vi "Configure Line Synchronization.vi"(6 "Enable Line Sync (F: Disable)":bool, 8 "error in (no error)":errorcluster, 9 "Channel List(\"\")":string, 10 "Function (0: Voltage DC)":i32(ring) items=[" Voltage DC"=0, "Current DC"=2, "Resistance"=4, "4-wire resistance"=5, "Temperature"=8, "Continuity"=9, "Voltage Ratio"=12], 11 "VISA resource name":refnum<visa-resource-name>) -> (0 "error out":errorcluster, 3 "VISA resource name out":refnum<visa-resource-name>)   [LabVIEW 2020, in "Keithley DMM6500 DAQ6500 Series.lvlib"]
doc: "Determines if line synchronization is used during the measurement."
uses:
  <instrlib>/Keithley DMM6500 DAQ6500 Series/Keithley DMM6500 DAQ6500 Series.lvlib
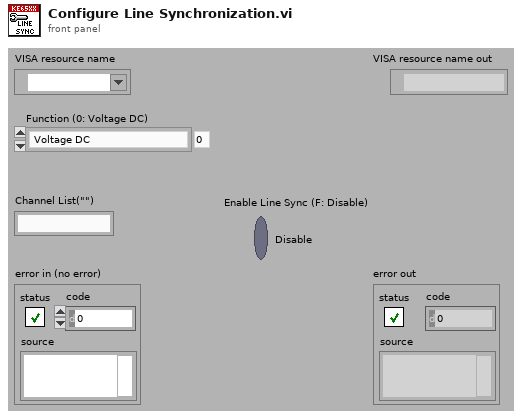
[diagram p1: front panel]
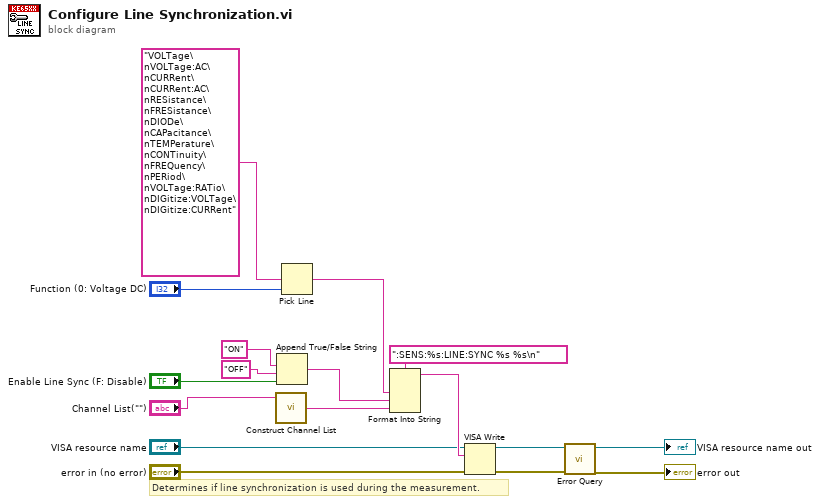
[diagram p0: block diagram]
diagram:
  # "Determines if line synchronization is used during the measurement."
  n1 = call <instrlib>:"Construct Channel List.vi"("Channel List"="Channel List(\"\")") -> ("Channel List String"=w2:string)  [unwired: 2 in]
  n2 = Append True/False String(1:"Enable Line Sync (F: Disable)", 2:"OFF", 3:"ON") -> (0:w14:string)  [unwired: 1 in]
  n3 = Pick Line(multi-line string="VOLTage\nVOLTage:AC\nCURRent\nCURRent:AC\nRESistance\nFRESistance\nDIODe\nCAPacitance\nTEMPerature\nCONTinuity\nFREQuency\nPERiod\nVOLTage:RATio\nDIGitize:VOLTage\nDIGitize:CURRent", line index="Function (0: Voltage DC)") -> (output string=w4:string)  [unwired: 1 in]
  n4 = Format Into String(format string=":SENS:%s:LINE:SYNC %s %s\n", w4, w14, w2) -> (resulting string=w13:string)  [unwired: 2 in, 1 out]
  n5 = VISA Write(VISA resource name="VISA resource name", write buffer=w13, error in (no error)="error in (no error)") -> (VISA resource name out=w10:refnum<visa-resource-name>, error out=w9:errorcluster)  [unwired: 1 out]
  n6 = call <instrlib>:"Error Query.vi"("error in (no error)"=w9, "VISA resource name"=w10) -> ("error out"=→"error out":errorcluster, "VISA resource name out"=→"VISA resource name out":refnum<visa-resource-name>)  [unwired: 6 in, 2 out]
